vi "publish status.vi"(8 "error in (no error)":errorcluster, 11 "S4ICS in":refnum<class "S4ICS.lvclass">) -> (0 "error out":errorcluster, 3 "S4ICS out":refnum<class "S4ICS.lvclass">)   [LabVIEW 2018, in "S4ICS.lvclass"]
uses:
  S4ICS.lvclass
  S4ICS.lvclass/S4ICS.ctl
  RxTx/RxTx.lvclass
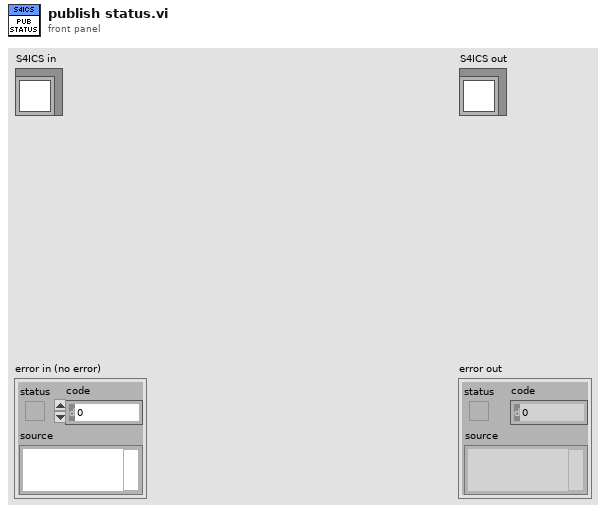
[diagram p1: front panel]
types:
  T1 = cluster{"broker":string, "version":string, "comment":string, "tcpServerSocket":string, "tcpServerEnabled":bool, "timestamp":string, "mechanisms":cluster{"name":string, "status":cluster{"mode":string, "condition":string, "position":string, "pos_name":string, "pos_id":string}}[]}
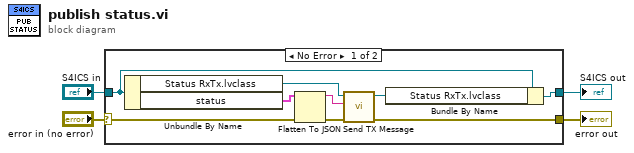
[diagram p0: block diagram]
diagram:
  n1 = case shown="No Error" "error in (no error)" {
    selector: "error in (no error)" -> [w6 w15]
    tunnel: [w12 w15] -> w3
    tunnel: [w8 w14] -> w1
    tunnel: "S4ICS in" -> [w9 w14]
    frame No Error {
      n2 = Unbundle By Name(w9) -> ("Status RxTx.lvclass"=w10:refnum<class "RxTx.lvclass">, "status"=w7:T1)
      n3 = Flatten To JSON(anything=w7, error in (no error)=w6) -> (JSON string=w5:string, 11:w11:errorcluster)  [unwired: 1 in]
      n4 = call "Send TX Message.vi"("error in (no error)"=w11, "element"=w5, "RxTx in"=w10) -> ("error out"=w12:errorcluster, "RxTx out"=w13:refnum<class "RxTx.lvclass">)  [unwired: 7 in]
      n5 = Bundle By Name(cluster=w9, "Status RxTx.lvclass"=w13) -> (w8:refnum<class "S4ICS.lvclass">)
    }
    frame Error {
    }
  }
  "error out" <- w3
  "S4ICS out" <- w1
